vi "Main.vi"(8 "error in":errorcluster, 11 "Spectro Acquisition in":refnum<class "Spectro Acquisition.lvclass">) -> (0 "error out":errorcluster, 3 "Spectro Acquisition out":refnum<class "Spectro Acquisition.lvclass">)   [LabVIEW 2024, in "Spectro Acquisition.lvclass"]
doc: "The <b>Queued Message Handler</b> of the Worker that owns this VI."
uses:
  Spectro Acquisition.lvclass
  Initialization Data.ctl
  Response Cases.ctl
  UI SmarAct/Data Queue.ctl
  Etat Acquisition Spectro.ctl
  Spectro Acquisition.lvclass/Spectro Acquisition.ctl
  rql_Acquisition en cours.ctl
  rqp_Start Acquisition.ctl
  rqp_Stop Acquisition.ctl
  rqp_Set Int Time.ctl
  rqp_Update Background.ctl
  rqp_Appliquer BKG.ctl
  rwr_One Acquisition.ctl
  rwr_One Acquisition Reply.ctl
  rqp_Init One Acquisition.ctl
  rqp_Appliquer calibration.ctl
  <vilib>/ErrorRing/Error Ring.xnode
  UI SmarAct/UI SmarAct.lvclass
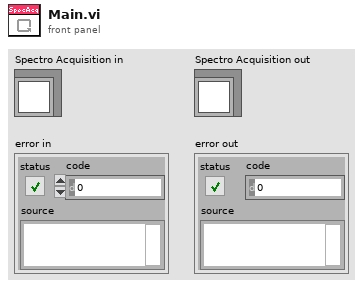
[diagram p1: front panel]
types:
  T1 = typedef "Spectro Acquisition.lvclass/Etat Acquisition Spectro.ctl" = enum16{"Veille", "En Acquisition", "Stop Acquisition", "One Acquisition"}
  T2 = typedef "Spectro Acquisition.lvclass/Initialization Data.ctl" = cluster{"Data Spectro":T3, "Data Queue":T4}
  T3 = typedef "Spectro Acquisition.lvclass/Response Cases.ctl" = cluster{"Placeholder - Can be deleted":string, "Wrapper Spectro":u32}
  T4 = typedef "UI SmarAct.lvclass/Data Queue.ctl" = cluster{"Queue Data":refnum<queue>}
  T5 = typedef "Spectro Acquisition.lvclass/rql_Acquisition en cours.ctl" = cluster{"String":string}
  T6 = typedef "Spectro Acquisition.lvclass/rqp_Start Acquisition.ctl" = cluster{"Wrapper Spectro":u32}
  T7 = typedef "Spectro Acquisition.lvclass/rqp_Stop Acquisition.ctl" = cluster{"String":string}
  T8 = typedef "Spectro Acquisition.lvclass/rqp_Set Int Time.ctl" = cluster{"Tps Int(ms)":u32}
  T9 = typedef "Spectro Acquisition.lvclass/rqp_Update Background.ctl" = cluster{"String":string}
  T10 = typedef "Spectro Acquisition.lvclass/rqp_Appliquer BKG.ctl" = cluster{"BackGround?":bool}
  T11 = typedef "Spectro Acquisition.lvclass/rwr_One Acquisition Reply.ctl" = cluster{"Spectre-BKG":dbl[], "Nbr de Scans":i32, "Spectrogramme One Acq":dbl[][]}
  T12 = typedef "Spectro Acquisition.lvclass/rwr_One Acquisition.ctl" = cluster{"Init Incr":i32}
  T13 = typedef "Spectro Acquisition.lvclass/rqp_Init One Acquisition.ctl" = cluster{"Init Incrément":i32}
  T14 = typedef "Spectro Acquisition.lvclass/rqp_Appliquer calibration.ctl" = cluster{"Calib?":bool}
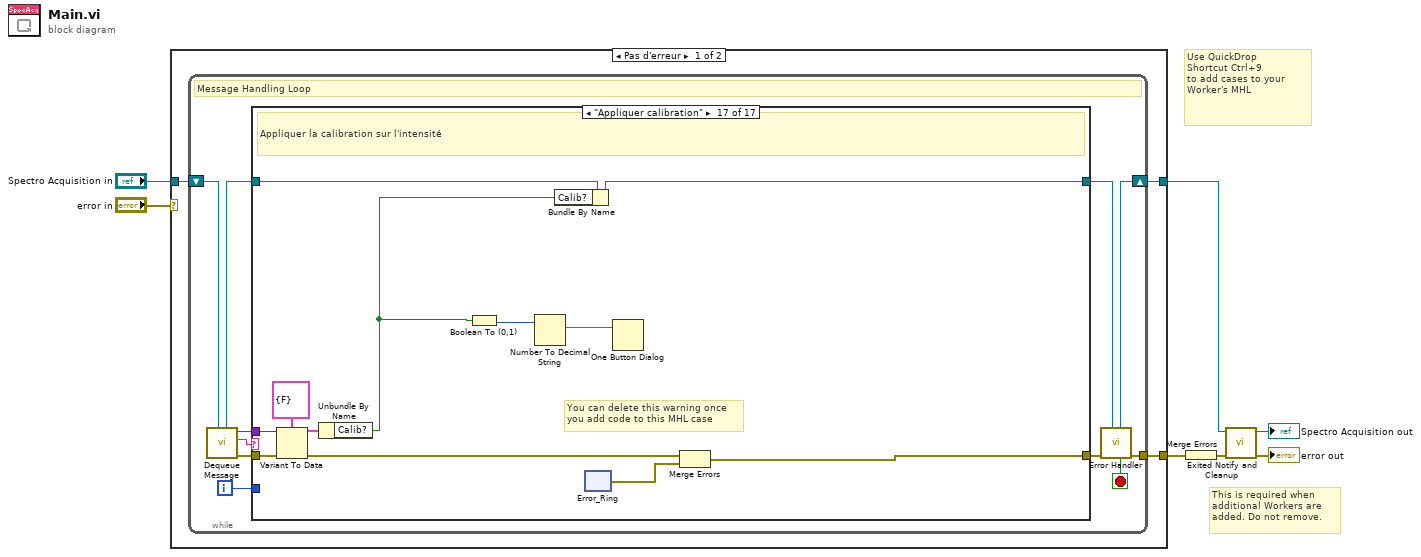
[diagram p0: block diagram]
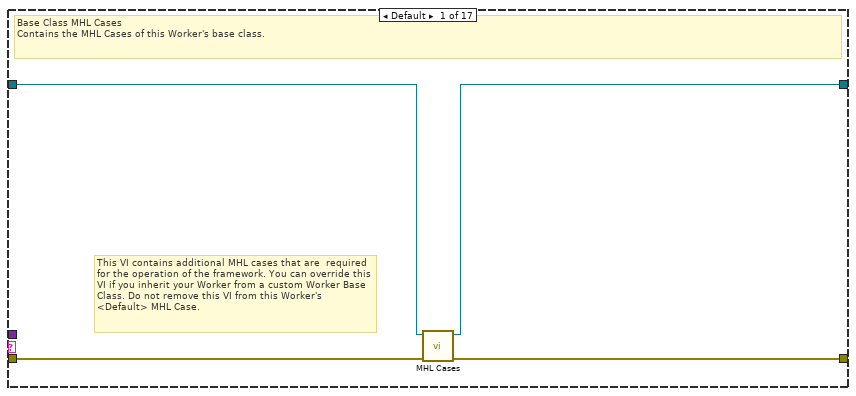
[diagram p2: hidden frame]
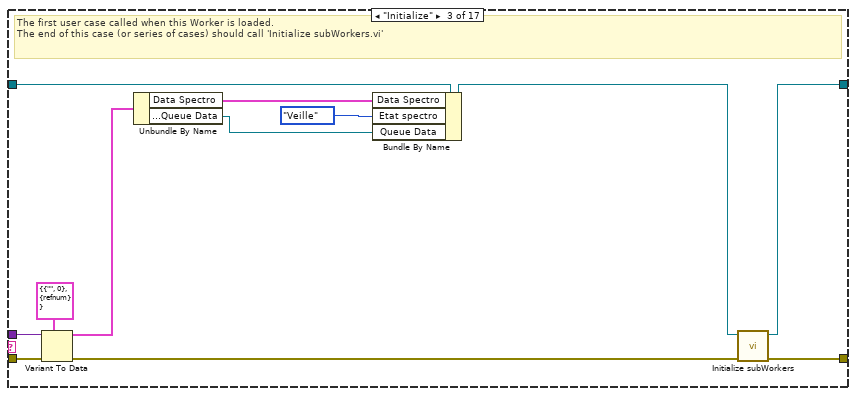
[diagram p4: hidden frame]
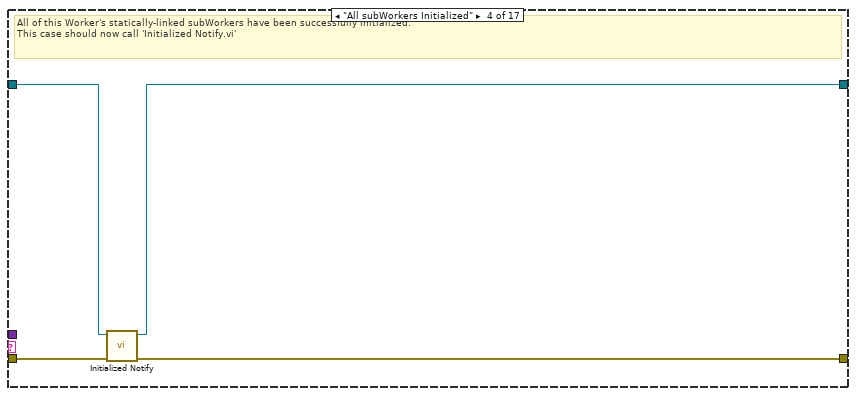
[diagram p5: hidden frame]
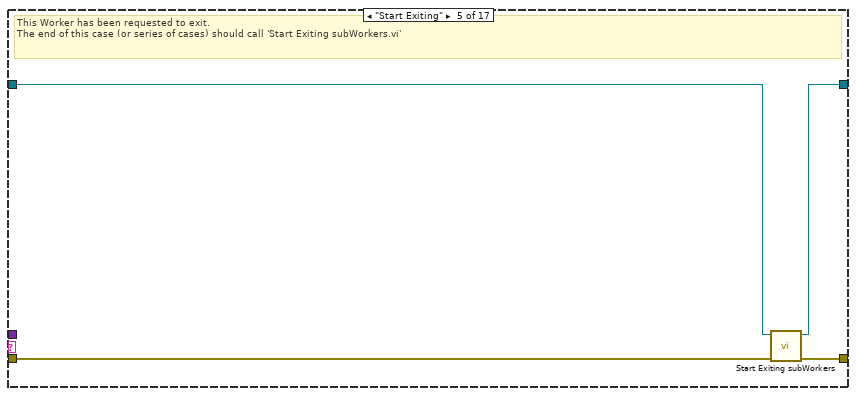
[diagram p6: hidden frame]
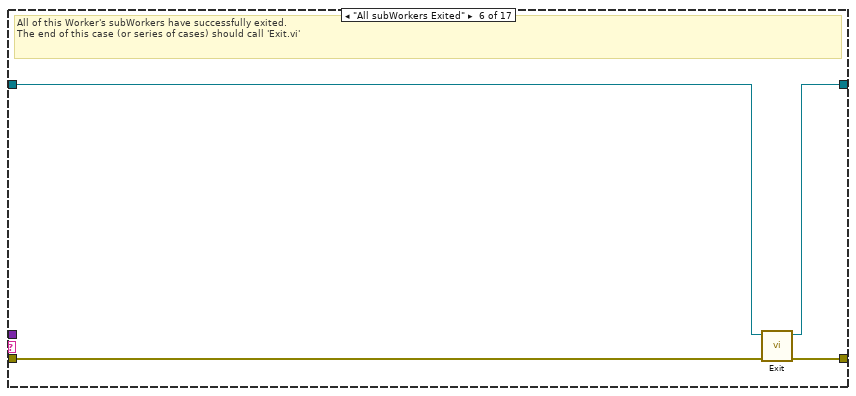
[diagram p7: hidden frame]
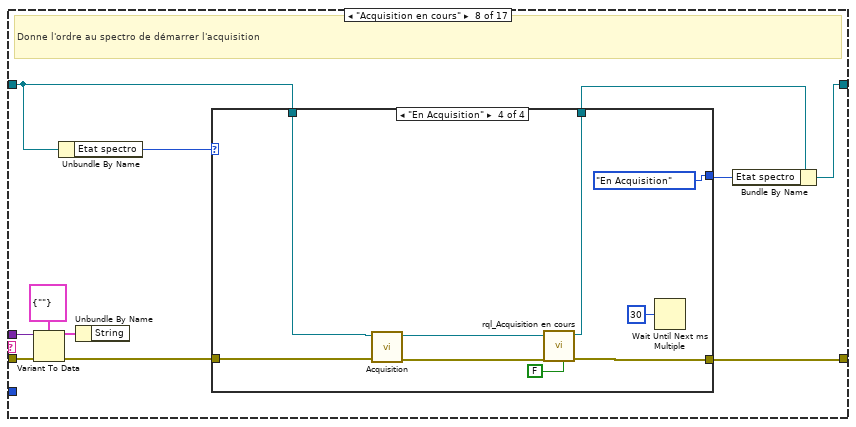
[diagram p9: hidden frame]
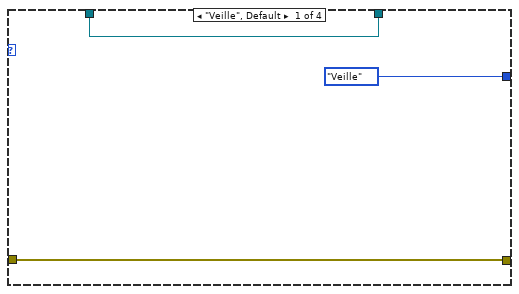
[diagram p10: hidden frame]
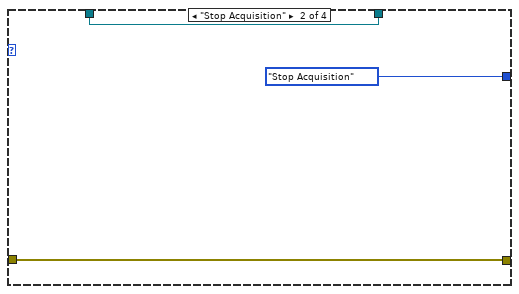
[diagram p11: hidden frame]
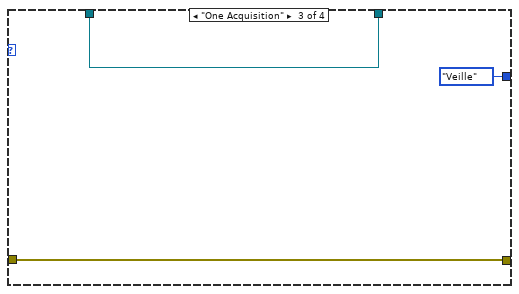
[diagram p12: hidden frame]
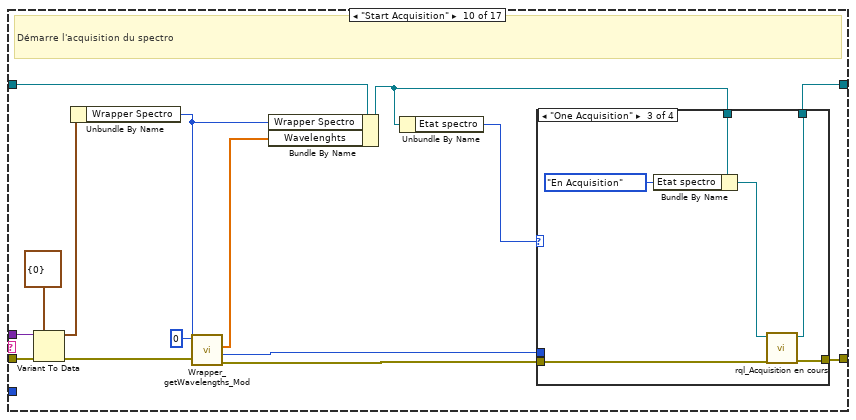
[diagram p14: hidden frame]
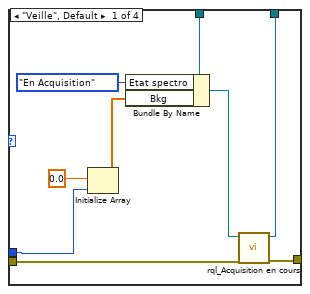
[diagram p15: hidden frame]
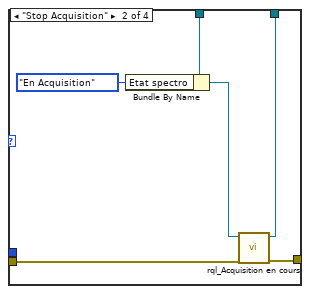
[diagram p16: hidden frame]
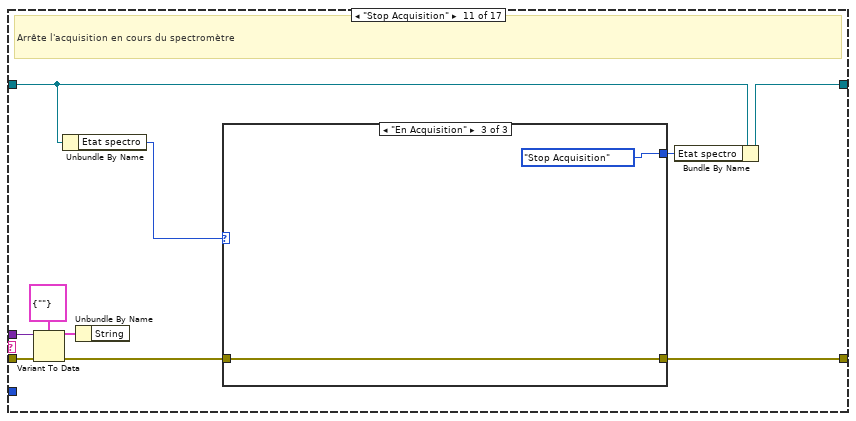
[diagram p18: hidden frame]
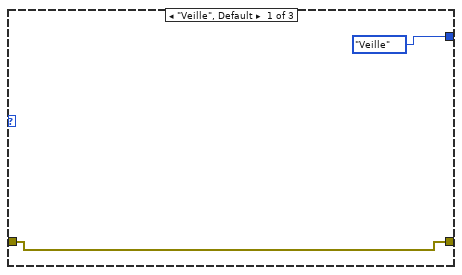
[diagram p19: hidden frame]
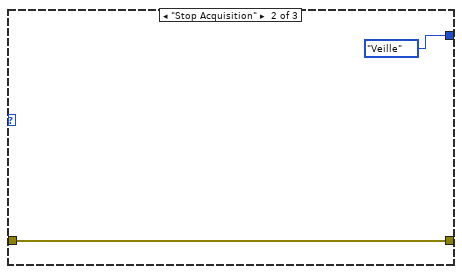
[diagram p20: hidden frame]
diagram:
  # "Use QuickDrop\nShortcut Ctrl+9\nto add cases to your\nWorker's MHL"
  # "This is required when additional Workers are added. Do not remove."
  n1 = case shown="Pas d'erreur" "error in" {
    tunnel: "Spectro Acquisition in" -> [w8 w217]
    tunnel: [w10 w218] -> w6
    tunnel: [w9 w216] -> w7
    selector: "error in" -> [_ w219]
    frame No Error {
      n2 = while {
        shift-right: [w19] -> w9
        shift-left: w8 -> [w21]
        tunnel: [w20] -> w10
        i -> [w12]
        stop <- w13 stop-if-true
        # "Message Handling Loop"
        n3 = call-dynamic "Dequeue Message.vi"("Worker"=w21) -> ("error out"=w18:errorcluster, "Case out"=w14:string, "Data out"=w11:variant, "Worker out"=w16:refnum<class "Spectro Acquisition.lvclass">)  [unwired: 6 in, 1 out]
        n4 = case "Worker MHL Case Structure (DO NOT CHANGE LABEL NAME)" shown="\"Appliquer calibration\"" w14 {
          tunnel: w18 -> [w25 w26 w37 w43 w44 w51 w53 w64 w84 w99 w132 w152 w160 w167 w187 w201 w213]
          tunnel: [w24 w26 w39 w42 w47 w50 w53 w56 w84 w95 w123 w145 w159 w166 w183 w200 w208] -> w17
          tunnel: w16 -> [w23 w27 w36 w41 w45 w49 w52 w55 w83 w93 w126 w148 w155 w168 w174 w202 w214]
          tunnel: [w22 w27 w38 w40 w46 w48 w52 w58 w83 w92 w128 w147 w154 w162 w182 w196 w206] -> w15
          tunnel: w12 -> [_ _ _ _ _ _ _ _ _ _ _ _ _ _ _ _ _]
          tunnel: w11 -> [_ _ w35 _ _ _ _ w62 _ w97 w130 w150 w157 w164 w185 w198 w210]
          frame Default {
            # "This VI contains additional MHL cases that are  required for the operation of the framework. You can override this VI if you inherit your Worker from a custom Worker Base Class. Do not remove this VI from this Worker's <Default> MHL Case."
            # "Base Class MHL Cases\nContains the MHL Cases of this Worker's base class."
            n5 = call-dynamic "MHL Cases.vi"("error in"=w25, "Worker in"=w23) -> ("error out"=w24:errorcluster, "Worker out"=w22:refnum<class "Spectro Acquisition.lvclass">)  [unwired: 8 in]
          }
          frame "------------ FRAMEWORK CASES -----------" {
            # "Start of Workers Framework Cases"
          }
          frame "Initialize" {
            # "The first user case called when this Worker is loaded.\nThe end of this case (or series of cases) should call 'Initialize subWorkers.vi'"
            n6 = Variant To Data(error in=w37, type=T2 {"Data Spectro"={"Placeholder - Can be deleted"="", "Wrapper Spectro"=0}, "Data Queue"={"Queue Data"=refnum}} ("Cluster"), Variant=w35) -> (data=w33:T2, error out=w29:errorcluster)
            n7 = Unbundle By Name(w33) -> ("Data Spectro"=w31:T3, "Data Queue.Queue Data"=w28:refnum<queue>)
            n8 = Bundle By Name(cluster=w36, "Data Spectro"=w31, "Etat spectro"=Etat_Acquisition_Spectro."Veille", "Queue Data"=w28) -> (w34:refnum<class "Spectro Acquisition.lvclass">)
            n9 = call-dynamic "Initialize subWorkers.vi"("error in"=w29, "Worker"=w34) -> ("error out"=w39:errorcluster, "dup Worker out"=w38:refnum<class "Spectro Acquisition.lvclass">)  [unwired: 8 in]
          }
          frame "All subWorkers Initialized" {
            # "All of this Worker's statically-linked subWorkers have been successfully initialized.\nThis case should now call 'Initialized Notify.vi'"
            n10 = call-dynamic "Initialized Notify.vi"("error in"=w43, "Worker"=w41) -> ("error out"=w42:errorcluster, "dup Worker out"=w40:refnum<class "Spectro Acquisition.lvclass">)  [unwired: 8 in]
          }
          frame "Start Exiting" {
            # "This Worker has been requested to exit. \nThe end of this case (or series of cases) should call 'Start Exiting subWorkers.vi'"
            n11 = call-dynamic "Start Exiting subWorkers.vi"("error_in"=w44, "Worker"=w45) -> ("error out"=w47:errorcluster, "dup Worker out"=w46:refnum<class "Spectro Acquisition.lvclass">)  [unwired: 8 in]
          }
          frame "All subWorkers Exited" {
            # "All of this Worker's subWorkers have successfully exited. \nThe end of this case (or series of cases) should call 'Exit.vi'"
            n12 = call-dynamic "Exit.vi"("error_in"=w51, "Worker"=w49) -> ("error out"=w50:errorcluster, "dup Worker out"=w48:refnum<class "Spectro Acquisition.lvclass">)  [unwired: 8 in]
          }
          frame "------------- LOCAL API CASES -------------" {
            # "Start of Workers Local API Cases"
          }
          frame "Acquisition en cours" {
            # "Donne l'ordre au spectro de démarrer l'acquisition"
            n13 = Variant To Data(error in=w64, type=T5 {"String"=""} ("Data"), Variant=w62) -> (data=w61:T5, error out=w59:errorcluster)
            n14 = Unbundle By Name(w55) -> ("Etat spectro"=w60:T1)
            n15 = Unbundle By Name(w61) -> ()  [unwired: 1 out]
            n16 = case shown="\"En Acquisition\"" w60 {
              tunnel: w59 -> [w65 w68 w73 w74]
              tunnel: [Etat_Acquisition_Spectro."Veille" ("Etat spectro") Etat_Acquisition_Spectro."Stop Acquisition" ("Etat spectro") Etat_Acquisition_Spectro."Veille" ("Etat spectro") Etat_Acquisition_Spectro."En Acquisition" ("Etat spectro")] -> w57
              tunnel: [w65 w68 w73 w80] -> w56
              tunnel: w55 -> [w66 w69 w72 w77]
              tunnel: [w66 w69 w72 w79] -> w54
              frame "Veille", Default {
              }
              frame "Stop Acquisition" {
              }
              frame "One Acquisition" {
              }
              frame "En Acquisition" {
                n17 = call "Acquisition.vi"("error in (no error)"=w74, "Spectro Acq en entrée"=w77) -> ("error out"=w75:errorcluster, "Spectro Acq en sortie"=w76:refnum<class "Spectro Acquisition.lvclass">)  [unwired: 8 in]
                n18 = call "rql_Acquisition en cours.vi"("Show in Debugger?"=FALSE, "error in"=w75, "Spectro Acquisition in"=w76) -> ("error out"=w80:errorcluster, "dup Spectro Acquisition out"=w79:refnum<class "Spectro Acquisition.lvclass">)  [unwired: 7 in]
                n19 = Wait Until Next ms Multiple(millisecond multiple=u32 30 ("attente (ms)")) -> ()  [unwired: 1 out]
              }
            }
            n20 = Bundle By Name(cluster=w54, "Etat spectro"=w57) -> (w58:refnum<class "Spectro Acquisition.lvclass">)
          }
          frame "------------- PUBLIC API CASES -------------" {
            # "Start of Workers Public API Cases"
          }
          frame "Start Acquisition" {
            # "Démarre l'acquisition du spectro"
            n21 = Variant To Data(error in=w99, type=T6 {"Wrapper Spectro"=0} ("Data"), Variant=w97) -> (data=w96:T6, error out=w90:errorcluster)
            n22 = Unbundle By Name(w96) -> ("Wrapper Spectro"=w88:u32)
            n23 = call "Wrapper_getWavelengths_Mod.vi"("error in (no error)"=w90, "Wrapper"=w88, "Index"=0) -> ("error out"=w89:errorcluster, "Length"=w85:i32, "WL Values"=w86:dbl[])  [unwired: 6 in]
            n24 = Bundle By Name(cluster=w93, "Wrapper Spectro"=w88, "Wavelenghts"=w86) -> (w91:refnum<class "Spectro Acquisition.lvclass">)
            n25 = Unbundle By Name(w91) -> ("Etat spectro"=w94:T1)
            n26 = case shown="\"One Acquisition\"" w94 {
              tunnel: [w105 w111 w117 w122] -> w95
              tunnel: w89 -> [w106 w112 w118 w122]
              tunnel: w91 -> [w108 w114 w120 w121]
              tunnel: [w103 w109 w115 w121] -> w92
              tunnel: w85 -> [w100 _ _ _]
              frame "Veille", Default {
                n27 = Initialize Array(0.0, w100) -> (w101:dbl[])
                n28 = Bundle By Name(cluster=w108, "Etat spectro"=Etat_Acquisition_Spectro."En Acquisition", "Bkg"=w101) -> (w104:refnum<class "Spectro Acquisition.lvclass">)
                n29 = call "rql_Acquisition en cours.vi"("error in"=w106, "Spectro Acquisition in"=w104) -> ("error out"=w105:errorcluster, "dup Spectro Acquisition out"=w103:refnum<class "Spectro Acquisition.lvclass">)  [unwired: 8 in]
              }
              frame "Stop Acquisition" {
                n30 = Bundle By Name(cluster=w114, "Etat spectro"=Etat_Acquisition_Spectro."En Acquisition") -> (w110:refnum<class "Spectro Acquisition.lvclass">)
                n31 = call "rql_Acquisition en cours.vi"("error in"=w112, "Spectro Acquisition in"=w110) -> ("error out"=w111:errorcluster, "dup Spectro Acquisition out"=w109:refnum<class "Spectro Acquisition.lvclass">)  [unwired: 8 in]
              }
              frame "One Acquisition" {
                n32 = Bundle By Name(cluster=w120, "Etat spectro"=Etat_Acquisition_Spectro."En Acquisition") -> (w116:refnum<class "Spectro Acquisition.lvclass">)
                n33 = call "rql_Acquisition en cours.vi"("error in"=w118, "Spectro Acquisition in"=w116) -> ("error out"=w117:errorcluster, "dup Spectro Acquisition out"=w115:refnum<class "Spectro Acquisition.lvclass">)  [unwired: 8 in]
              }
              frame "En Acquisition" {
              }
            }
          }
          frame "Stop Acquisition" {
            # "Arrête l'acquisition en cours du spectromètre"
            n34 = Variant To Data(error in=w132, type=T7 {"String"=""} ("Data"), Variant=w130) -> (data=w129:T7, error out=w127:errorcluster)
            n35 = Unbundle By Name(w126) -> ("Etat spectro"=w125:T1)
            n36 = Unbundle By Name(w129) -> ()  [unwired: 1 out]
            n37 = case shown="\"En Acquisition\"" w125 {
              tunnel: w127 -> [w133 w135 w137]
              tunnel: [Etat_Acquisition_Spectro."Veille" ("Etat spectro") Etat_Acquisition_Spectro."Veille" ("Etat spectro") Etat_Acquisition_Spectro."Stop Acquisition" ("Etat spectro")] -> w124
              tunnel: [w133 w135 w137] -> w123
              frame "Veille", Default {
              }
              frame "Stop Acquisition" {
              }
              frame "En Acquisition" {
              }
            }
            n38 = Bundle By Name(cluster=w126, "Etat spectro"=w124) -> (w128:refnum<class "Spectro Acquisition.lvclass">)
          }
          frame "Set Int Time" {
            # "Mise à jour du temps d'intégration"
            n39 = Variant To Data(error in=w152, type=T8 {"Tps Int(ms)"=0} ("Data"), Variant=w150) -> (data=w149:T8, error out=w146:errorcluster)
            n40 = Unbundle By Name(w149) -> ("Tps Int(ms)"=w140:u32)
            n41 = Unbundle By Name(w148) -> ("Wrapper Spectro"=w142:u32)
            n42 = Multiply(x=w140, y=u32 1000) -> (x*y=w139:u32)
            n43 = call "Wrapper_setIntegrationTime_Mod.vi"("error in (no error)"=w146, "Integration Time"=w139, "Wrapper In"=w142, "Index"=0) -> ("error out"=w145:errorcluster, "Wrapper Out"=w144:u32)  [unwired: 6 in]
            n44 = Bundle By Name(cluster=w148, "Wrapper Spectro"=w144) -> (w147:refnum<class "Spectro Acquisition.lvclass">)
          }
          frame "Update Background" {
            # "Fait le bruit de fond"
            n45 = Variant To Data(error in=w160, type=T9 {"String"=""} ("Data"), Variant=w157) -> (data=w156:T9, error out=w159:errorcluster)
            n46 = Unbundle By Name(w156) -> ()  [unwired: 1 out]
            n47 = Unbundle By Name(w155) -> ("Spectre Brut"=w153:dbl[])
            n48 = Bundle By Name(cluster=w155, "Bkg"=w153) -> (w154:refnum<class "Spectro Acquisition.lvclass">)
          }
          frame "Appliquer BKG" {
            # "Apliquer la soustraction du bruit de fond"
            n49 = Variant To Data(error in=w167, type=T10 {"BackGround?"=FALSE} ("Data"), Variant=w164) -> (data=w163:T10, error out=w166:errorcluster)
            n50 = Unbundle By Name(w163) -> ("BackGround?"=w161:bool)
            n51 = Bundle By Name(cluster=w168, "BackGround?"=w161) -> (w162:refnum<class "Spectro Acquisition.lvclass">)
          }
          frame "One Acquisition" {
            # "Scan avec une acquisition du spectro"
            n52 = Variant To Data(error in=w187, type=T12 {"Init Incr"=0} ("Data"), Variant=w185) -> (data=w184:T12, error out=w179:errorcluster)
            n53 = Unbundle By Name(w174) -> ("Init Incrément"=w173:i32)
            n54 = Unbundle By Name(w184) -> ()  [unwired: 1 out]
            n55 = disable-structure shown="Activé" {
              disable-tunnel: w179 -> [w191 w193]
              disable-tunnel: [w190 w193] -> w178
              disable-tunnel: w174 -> [w189 w192]
              disable-tunnel: [w188 w192] -> w177
              frame Enabled {
                n56 = call "Acquisition.vi"("error in (no error)"=w191, "Spectro Acq en entrée"=w189) -> ("error out"=w190:errorcluster, "Spectro Acq en sortie"=w188:refnum<class "Spectro Acquisition.lvclass">)  [unwired: 8 in]
              }
              frame Disabled {
              }
            }
            n57 = Unbundle By Name(w177) -> ("Spectrogramme One Acq"=w171:dbl[][], "Spectre-BKG"=w169:dbl[])
            n58 = Increment(x=w173) -> (x+1=w172:i32)
            n59 = Build Array (concatenate)(w171, w169) -> (w170:dbl[][])
            n60 = Bundle By Name(cluster=T11 {"Spectre-BKG"=[], "Nbr de Scans"=0, "Spectrogramme One Acq"=[]} ("Reply Data"), "Spectrogramme One Acq"=w170, "Spectre-BKG"=w169, "Nbr de Scans"=w172) -> (w180:T11)
            n61 = Bundle By Name(cluster=w177, "Etat spectro"=Etat_Acquisition_Spectro."One Acquisition", "Init Incrément"=w172, "Spectrogramme One Acq"=w170) -> (w176:refnum<class "Spectro Acquisition.lvclass">)
            n62 = call-dynamic "Callback Easy Reply.vi"("error in"=w178, "Data"=w180, "Worker"=w176) -> ("error out"=w183:errorcluster, "dup Worker out"=w182:refnum<class "Spectro Acquisition.lvclass">)  [unwired: 7 in]
          }
          frame "Init One Acquisition" {
            # "Initialise l'acquisition"
            n63 = Variant To Data(error in=w201, type=T13 {"Init Incrément"=0} ("Data"), Variant=w198) -> (data=w197:T13, error out=w200:errorcluster)
            n64 = Unbundle By Name(w197) -> ("Init Incrément"=w195:i32)
            n65 = Bundle By Name(cluster=w202, "Init Incrément"=w195, "Spectrogramme One Acq"=dbl[][] []) -> (w196:refnum<class "Spectro Acquisition.lvclass">)
          }
          frame "Appliquer calibration" {
            # "You can delete this warning once\nyou add code to this MHL case"
            # "Appliquer la calibration sur l'intensité"
            n66 = Variant To Data(error in=w213, type=T14 {"Calib?"=FALSE} ("Data"), Variant=w210) -> (data=w209:T14, error out=w212:errorcluster)
            n67 = Unbundle By Name(w209) -> ("Calib?"=w205:bool)
            n68 = Boolean To (0,1)(Boolean=w205) -> (0, 1=w204:i16)
            n69 = Number To Decimal String(number=w204) -> (decimal integer string=w203:string)  [unwired: 1 in]
            n70 = Bundle By Name(cluster=w214, "Calib?"=w205) -> (w206:refnum<class "Spectro Acquisition.lvclass">)
            n71 = xnode ("Error_Ring")() -> ("sortie d'erreur"=w207:errorcluster)
            n72 = One Button Dialog(message=w203) -> ()  [unwired: 1 in, 1 out]
            n73 = Merge Errors(w212, w207) -> (w208:errorcluster)
          }
        }
        n74 = call-dynamic "Error Handler.vi"("Worker"=w15, "error_in"=w17) -> ("error out"=w20:errorcluster, "Stop Loop"=w13:bool, "Worker out"=w19:refnum<class "Spectro Acquisition.lvclass">)  [unwired: 7 in]
      }
    }
    frame Error {
      n75 = call-dynamic "Error Handler.vi"("Worker"=w217, "error_in"=w219) -> ("error out"=w218:errorcluster, "Worker out"=w216:refnum<class "Spectro Acquisition.lvclass">)  [unwired: 7 in, 1 out]
    }
  }
  n76 = Merge Errors(w6) -> (w3:errorcluster)
  n77 = call-dynamic "Exited Notify and Cleanup.vi"("error_in"=w3, "Worker"=w7) -> ("error out"=→"error out":errorcluster, "dup Worker out"=→"Spectro Acquisition out":refnum<class "Spectro Acquisition.lvclass">)  [unwired: 8 in]
